vi "Approx Equal (1D-Scalar).vi"(4 "Y":dbl, 5 "X":dbl[](array[numeric])) -> (1 "X approx Y?":bool[](array[boolean]))   [LabVIEW 2020]
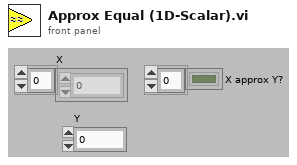
[diagram p1: front panel]
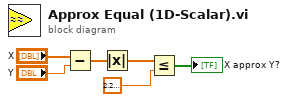
[diagram p0: block diagram]
diagram:
  n1 = Subtract(x="X", y="Y") -> (x-y=w4:dbl[])
  n2 = Absolute Value(x=w4) -> (abs(x)=w3:dbl[])
  n3 = Less Or Equal?(x=w3, y=2.220446049250313e-16) -> (x <= y?=→"X approx Y?":bool[])
